vi "Apply Steering Frame Velocity to Single Wheel.vi"(5 "constraint error tolerance (1E-12)":dbl=1e-12, 6 "apply data to motors":bool, 7 "wheel index":i32, 8 "error in (no error)":errorcluster, 9 "steering frame velocity":dbl[](array[numeric]), 11 "steering frame in":refnum<class "NI_Robotics_Steering Frame.lvclass">) -> (0 "error out":errorcluster, 3 "steering frame out":refnum<class "NI_Robotics_Steering Frame.lvclass">)   [LabVIEW 2017, in "NI_Robotics_Steering Frame.lvclass"]
uses:
  <vilib>/robotics/Steering/Steering Frame/NI_Robotics_Steering Frame.lvclass
  <vilib>/robotics/Steering/Steering Frame/NI_Robotics_Steering Frame.lvclass/NI_Robotics_Steering Frame.ctl
  <vilib>/robotics/Steering/Wheel/NI_Robotics_Wheel.lvclass/NI_Robotics_Wheel.ctl
  <vilib>/Analysis/baseanly.llb/A x Vector.vi
  <vilib>/robotics/Steering/Wheel/NI_Robotics_Wheel.lvclass
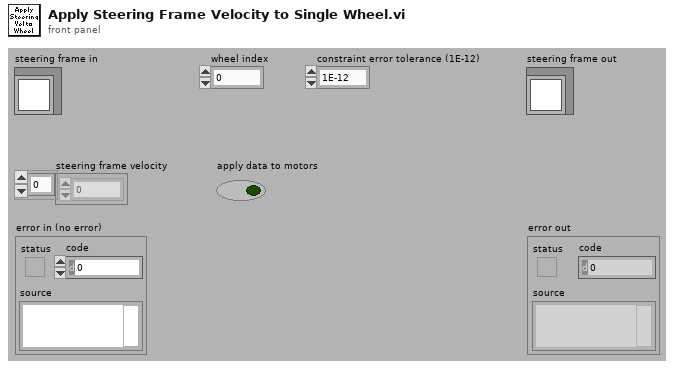
[diagram p1: front panel]
types:
  T1 = typedef "NI_Robotics_Wheel.lvclass/Wheel State.ctl" = cluster{"wheel name":string, "forward angular velocity":dbl, "caster angular velocity":dbl, "caster wheel angle (rad)":dbl, "steering angle (rad)":dbl}
  T2 = typedef "NI_Robotics_Steering Frame.lvclass/Wheel Orientation.ctl" = cluster{"wheel":refnum<class "NI_Robotics_Wheel.lvclass">, "x position":dbl, "y position":dbl, "frame angle (rad)":dbl}
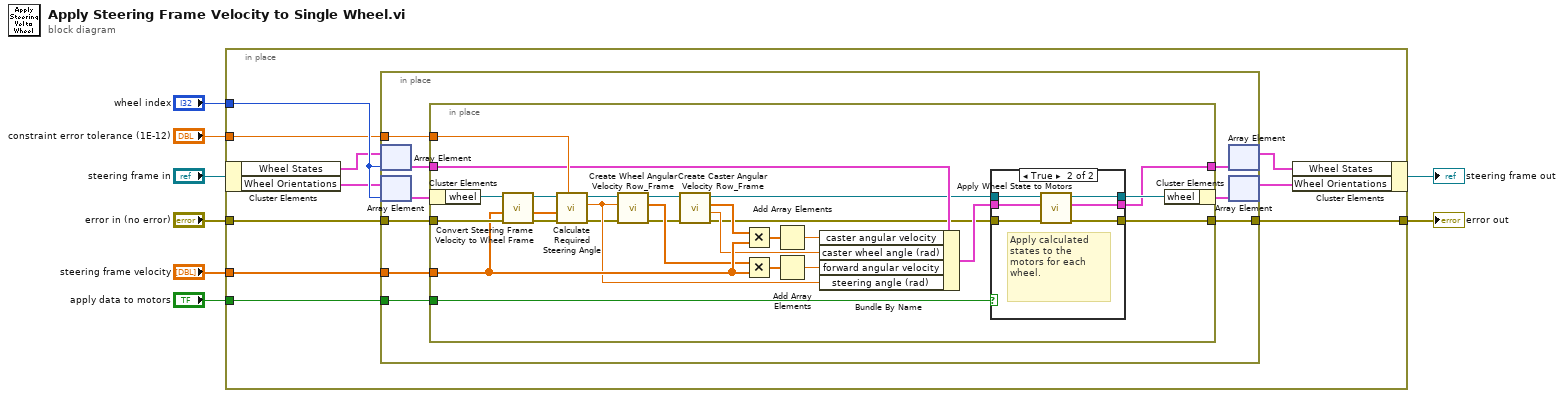
[diagram p0: block diagram]
diagram:
  n1 = in-place {
    in-place-border: "wheel index" -> [w18]
    in-place-border: "error in (no error)" -> [w17]
    in-place-border: "steering frame velocity" -> [w16]
    in-place-border: "apply data to motors" -> [w15]
    in-place-border: [w14] -> w4
    in-place-border: "constraint error tolerance (1E-12)" -> [w13]
    n2 = in-place-cluster #1("steering frame in") -> ("Wheel States"=w12:T1[], "Wheel Orientations"=w11:T2[])
    n3 = in-place {
      in-place-border: w13 -> [w27]
      in-place-border: w16 -> [w26]
      in-place-border: w17 -> [w25]
      in-place-border: [w24] -> w14
      in-place-border: w15 -> [w23]
      n4 = in-place-array #2(w12, w18) -> (w22:T1)
      n5 = in-place-array #3(w11, w18) -> (w20:T2)
      n6 = in-place {
        in-place-border: w27 -> [w53]
        in-place-border: w26 -> [w46]
        in-place-border: w25 -> [w51]
        in-place-border: [w43] -> w24
        in-place-border: w23 -> [w40]
        in-place-border: w22 -> [w45]
        in-place-border: [w41] -> w21
        n7 = in-place-cluster #4(w20) -> ("wheel"=w50:refnum<class "NI_Robotics_Wheel.lvclass">)
        n8 = call <vilib>:"Convert Steering Frame Velocity to Wheel Frame.vi"("error in (no error)"=w51, "steering frame velocity"=w46, "wheel in"=w50) -> ("error out"=w54:errorcluster, "wheel frame velocity"=w52:dbl[], "wheel out"=w49:refnum<class "NI_Robotics_Wheel.lvclass">)  [unwired: 6 in]
        n9 = call-dynamic "Calculate Required Steering Angle.vi"("constraint error tolerance (1E-12)"=w53, "error in (no error)"=w54, "wheel frame velocity"=w52, "wheel in"=w49) -> ("error out"=w28:errorcluster, "required steering angle (rad)"=w30:dbl, "wheel out"=w29:refnum<class "NI_Robotics_Wheel.lvclass">)  [unwired: 5 in]
        n10 = call <vilib>:"Create Wheel Angular Velocity Row_Frame.vi"("error in (no error)"=w28, "steering angle (rad)"=w30, "wheel in"=w29) -> ("error out"=w31:errorcluster, "wheel angular velocity row"=w33:dbl[], "wheel out"=w32:refnum<class "NI_Robotics_Wheel.lvclass">)  [unwired: 6 in]
        n11 = call <vilib>:"Create Caster Angular Velocity Row_Frame.vi"("error in (no error)"=w31, "wheel in"=w32) -> ("error out"=w34:errorcluster, "current caster angle"=w36:dbl, "wheel caster angular velocity row"=w37:dbl[], "wheel out"=w35:refnum<class "NI_Robotics_Wheel.lvclass">)  [unwired: 6 in]
        n12 = Multiply(x=w37, y=w46) -> (x*y=w47:dbl[])
        n13 = Multiply(x=w33, y=w46) -> (x*y=w48:dbl[])
        n14 = Add Array Elements(numeric array=w47) -> (sum=w39:dbl)
        n15 = Add Array Elements(numeric array=w48) -> (sum=w38:dbl)
        n16 = Bundle By Name(cluster=w45, "caster angular velocity"=w39, "caster wheel angle (rad)"=w36, "forward angular velocity"=w38, "steering angle (rad)"=w30) -> (w42:T1)
        n17 = case shown="True" w40 {
          tunnel: w34 -> [w55 w59]
          tunnel: [w55 w58] -> w43
          tunnel: w35 -> [w57 w63]
          tunnel: w42 -> [w56 w61]
          tunnel: [w56 w60] -> w41
          tunnel: [w57 w62] -> w44
          frame False {
          }
          frame True {
            # "Apply calculated states to the motors for each wheel."
            n18 = call <vilib>:"Apply Wheel State to Motors.vi"("error in (no error)"=w59, "wheel state in"=w61, "wheel in"=w63) -> ("error out"=w58:errorcluster, "wheel state out"=w60:T1, "wheel out"=w62:refnum<class "NI_Robotics_Wheel.lvclass">)  [unwired: 6 in]
          }
        }
        n19 = in-place-cluster #4("wheel"=w44) -> (w19:T2)
      }
      n20 = in-place-array #2(w21) -> (w10:T1[])  [unwired: 1 out]
      n21 = in-place-array #3(w19) -> (w9:T2[])  [unwired: 1 out]
    }
    n22 = in-place-cluster #1("Wheel States"=w10, "Wheel Orientations"=w9) -> (→"steering frame out":refnum<class "NI_Robotics_Steering Frame.lvclass">)
  }
  "error out" <- w4
